vi "SpectrumToColor.vi"(1 "Reflectance":dbl[](array[numeric]), 2 "CMF":dbl[][](array[numeric]), 3 "Illuminant":cluster{"String":string, "Array":dbl[]}, 4 "Selected RGB":string(combo)) -> (0 "Color,XYZ,RGB,Lab":T1)   [LabVIEW 2013]
panel:
  out "RGBStandardRows":i32
  out "RGBStandards":string[][](array[string])
  out "WhiteReference":i32[](array[numeric])
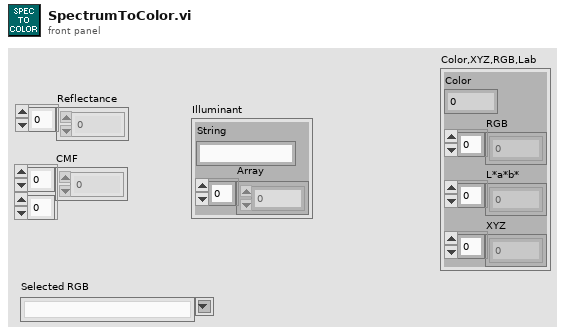
[diagram p1: front panel]
types:
  T1 = cluster{"Color":u32, "RGB":dbl[], "L*a*b*":dbl[], "XYZ":dbl[]}
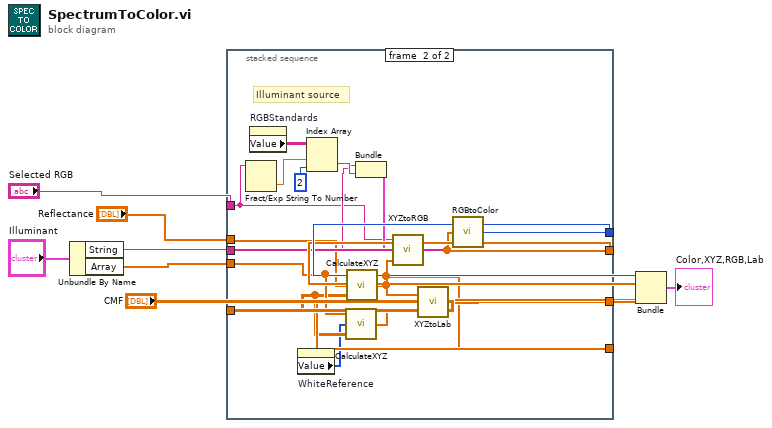
[diagram p0: block diagram]
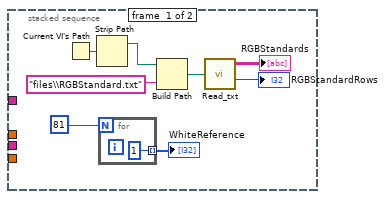
[diagram p2: hidden frame]
diagram:
  n1 = Unbundle By Name("Illuminant") -> ("String"=w1:string, "Array"=w2:dbl[])
  n2 = stacked-sequence {
    tunnel: w2 -> [_ w36]
    tunnel: "CMF" -> [_ w35]
    tunnel: [_ w32] -> w8
    tunnel: "Selected RGB" -> [_ w21]
    tunnel: [_ w31] -> w9
    tunnel: [_ w30] -> w10
    tunnel: [_ w29] -> w6
    tunnel: "Reflectance" -> [_ w28]
    tunnel: w1 -> [_ w22]
    frame #0 {
      n3 = Current VI's Path() -> (path=w14:path)
      n4 = Strip Path(path=w14) -> (stripped path=w13:path)  [unwired: 1 out]
      n5 = for {
        N: 81 -> [_]
        tunnel: [1] -> w19 mode=indexing
      }
      "WhiteReference" <- w19
      n6 = Build Path(base path=w13, name or relative path="files\\RGBStandard.txt") -> (appended path=w12:path)
      n7 = call "Read_txt.vi"("file path (dialog if empty)"=w12) -> ("Elements"=→"RGBStandards":string[][], "Rows"=→"RGBStandardRows":i32)  [unwired: 1 out]
    }
    frame #1 {
      # "Illuminant source"
      n8 = Fract/Exp String To Number(string=w21) -> (number=w25:dbl)  [unwired: 3 in, 1 out]
      n9 = property on="RGBStandards" class="Arr (strict)"() -> ("Value"=w27:string[][])  [unwired: 2 in, 2 out]
      n10 = property on="WhiteReference" class="Arr (strict)"() -> ("Value"=w34:i32[])  [unwired: 2 in, 2 out]
      n11 = Index Array(array=w27, index (row)=w25, index (col)=2 ("disabled index (col)")) -> (element=w23:string)
      n12 = call "CalculateXYZ.vi"("CMF"=w35, "Reflectance"=w34, "Illuminant"=w36) -> ("XYZ"=w33:dbl[])
      n13 = call "CalculateXYZ.vi"("CMF"=w35, "Reflectance"=w28, "Illuminant"=w36) -> ("XYZ"=w29:dbl[])
      n14 = Bundle("String"=w22, "String"=w23) -> (w24:cluster{"String":string, "String":string})  [unwired: 1 in]
      n15 = call "XYZtoRGB.vi"("XYZ"=w29, "Illuminants"=w24, "Selected RGB"=w21) -> ("RGB"=w31:dbl[])
      n16 = call "XYZtoLab.vi"("XrYrZr"=w33, "XYZ"=w29) -> ("L*a*b*"=w32:dbl[])
      n17 = call "RGBtoColor.vi"("RGB"=w31) -> ("Color"=w30:u32)
    }
  }
  n18 = Bundle("Color"=w10, "RGB"=w9, "L*a*b*"=w8, "XYZ"=w6) -> (→"Color,XYZ,RGB,Lab":T1)  [unwired: 1 in]
